vi "Exp_GetTemplate.vi"(8 "error in (no error)":errorcluster, 11 "LightField Automation in":refnum<class "LightField Automation.lvclass">) -> (0 "error out":errorcluster, 2 "Setting":i32, 3 "LightField Automation out":refnum<class "LightField Automation.lvclass">)   [LabVIEW 2015, in "LightField Automation.lvclass"]
uses:
  LightField Automation.lvclass
  C:/Program Files/Princeton Instruments/LightField/PrincetonInstruments.LightFieldAddInSupportServices.dll
  Program Files/Princeton Instruments/LightField/PrincetonInstruments.LightFieldAddInSupportServices.dll
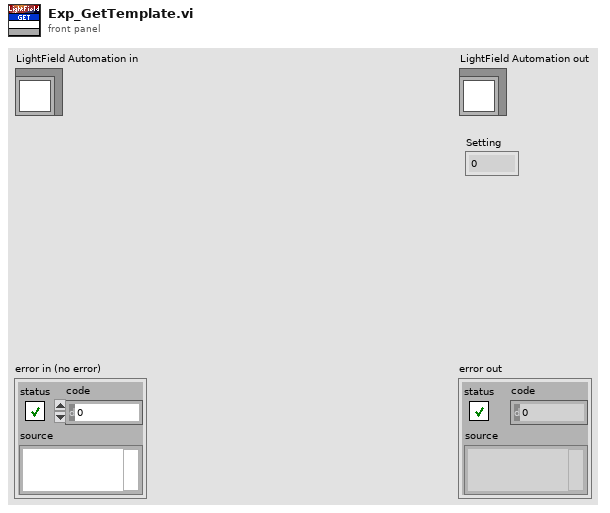
[diagram p1: front panel]
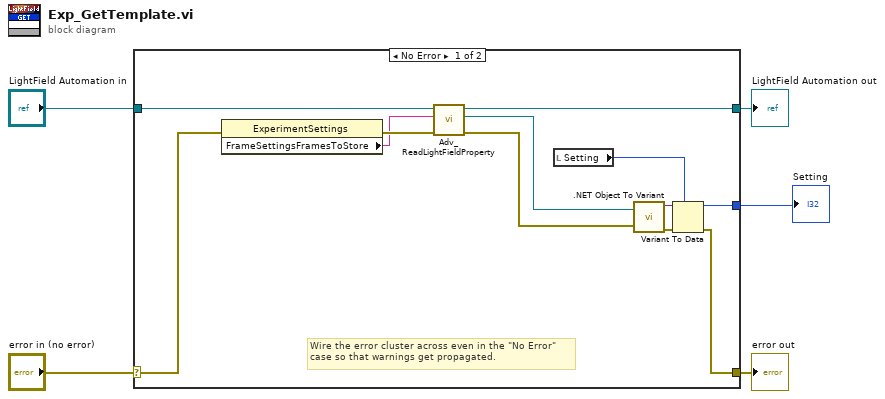
[diagram p0: block diagram]
diagram:
  n1 = case shown="No Error" "error in (no error)" {
    selector: "error in (no error)" -> [w15 w19]
    tunnel: [w13 w19] -> w4
    tunnel: [w10 w18] -> w2
    tunnel: "LightField Automation in" -> [w11 w18]
    tunnel: [w14 _] -> w1
    frame No Error {
      # "Wire the error cluster across even in the \"No Error\"\ncase so that warnings get propagated."
      n2 = property class="ExperimentSettings"(error in=w15) -> (error out=w9:errorcluster, "FrameSettingsFramesToStore"=w8:string)  [unwired: 1 in, 1 out]
      n3 = call "Adv_ReadLightFieldProperty.vi"("error in (no error)"=w9, "setting"=w8, "LightField Automation in"=w11) -> ("error out"=w6:errorcluster, "value"=w7:refnum<k24>, "LightField Automation out"=w10:refnum<class "LightField Automation.lvclass">)  [unwired: 6 in]
      n4 = local read "Setting"() -> (w12:i32)
      n5 = call <vilib>:".NET Object To Variant.vi"("error in (no error)"=w6, ".NET object"=w7) -> ("error out"=w17:errorcluster, "variant"=w16:variant)
      n6 = Variant To Data(error in=w17, type=w12, Variant=w16) -> (data=w14:i32, error out=w13:errorcluster)
    }
    frame Error {
    }
  }
  "error out" <- w4
  "LightField Automation out" <- w2
  "Setting" <- w1
